vi "TLPM VXIpnp Error Converter2.vi"(8 "error in (no error)":errorcluster {"code" format="%.0x"}, 9 "Name Of VI (\"\")":string, 10 "CVI Error Code (0)":i32 format="%.0x", 11 "instrument handle":u32) -> (0 "error out":errorcluster {"code" format="%.0x"}, 3 "instrument handle out":u32)   [LabVIEW 2023, in "Thorlabs Power Meter.lvlib"]
doc: "This VI converts error codes from VXIPnp instrument driver to standard LabVIEW error codes. If an error is detected the VI builds the appropriate error cluster that is readable by one of the error handlers supplied with LabVIEW."
uses:
  Thorlabs Power Meter.lvlib
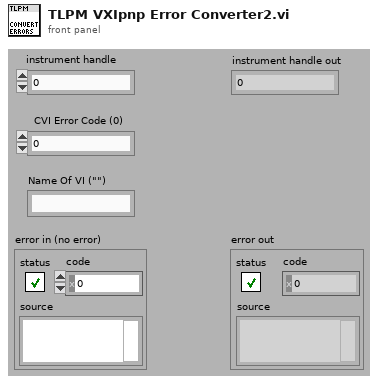
[diagram p1: front panel]
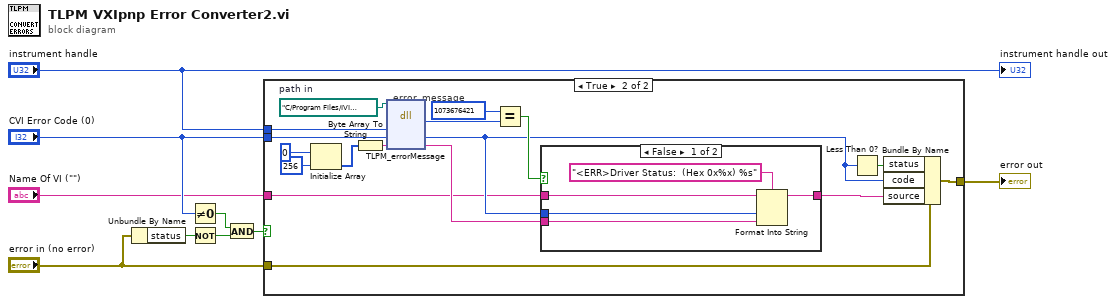
[diagram p0: block diagram]
diagram:
  n1 = Unbundle By Name("error in (no error)") -> ("status"=w8:bool)
  n2 = Not Equal To 0?(x="CVI Error Code (0)") -> (x != 0?=w9:bool)
  n3 = Not(x=w8) -> (.not. x?=w6:bool)
  n4 = And(x=w9, y=w6) -> (x .and. y?=w7:bool)
  n5 = case shown="True" w7 {
    tunnel: "CVI Error Code (0)" -> [_ w27]
    tunnel: [w10 w26] -> w4
    tunnel: "error in (no error)" -> [w10 w25]
    tunnel: "instrument handle" -> [_ w20]
    tunnel: "Name Of VI (\"\")" -> [_ w12]
    frame False {
    }
    frame True {
      w11 = path "C:/Program Files/IVI Foundation/VISA/Win64/Bin/TLPM_64.dll"  # path in
      # "error_message"
      n6 = Initialize Array(u8 0, 256) -> (w23:u8[])
      n7 = Byte Array To String(unsigned byte array=w23) -> (string=w21:string)
      n8 = dll-call lib="TLPM_64.dll" fn="TLPM_errorMessage"(path in=w11, w20, w27, w21) -> ("return type"=w18:i32, w13:i32, w16:string)  [unwired: 3 in, 2 out]
      n9 = Equal?(x=1073676421 ("y"), y=w18) -> (x = y?=w17:bool)
      n10 = case shown="False" w17 {
        tunnel: w16 -> [w30 _]
        tunnel: w12 -> [w32 w33]
        tunnel: w13 -> [w31 _]
        tunnel: [w29 w33] -> w15
        frame False {
          n11 = Format Into String(format string="<ERR>Driver Status:  (Hex 0x%x) %s", initial string=w32, w31, w30) -> (resulting string=w29:string)  [unwired: 1 in, 1 out]
        }
        frame True {
        }
      }
      n12 = Less Than 0?(x=w13) -> (x < 0?=w14:bool)
      n13 = Bundle By Name(cluster=w25, "status"=w14, "code"=w13, "source"=w15) -> (w26:errorcluster)
    }
  }
  "error out" <- w4
  "instrument handle out" <- "instrument handle"
